vi "Var_serrure2.vi"() -> ()   [LabVIEW 2018]
panel:
  in  "MAX":dbl=5.0
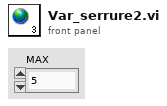
[diagram p1: front panel]
diagram:
